vi "SendWait.vi"(0 "session in":refnum<k35>, 5 "Time (s)":i32, 7 "Text To Wait":string, 11 "error in":errorcluster) -> (4 "session out":refnum<k35>, 15 "error out":errorcluster)   [LabVIEW 2023]
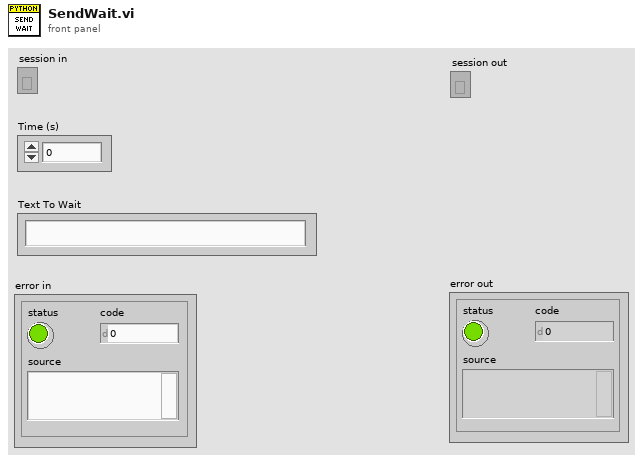
[diagram p1: front panel]
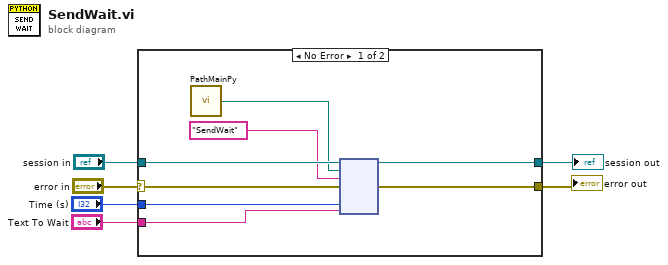
[diagram p0: block diagram]
diagram:
  n1 = case shown="No Error" "error in" {
    selector: "error in" -> [w11 w15]
    tunnel: "session in" -> [w14 w16]
    tunnel: [w13 w16] -> w3
    tunnel: [w12 w15] -> w4
    tunnel: "Text To Wait" -> [w8 _]
    tunnel: "Time (s)" -> [w7 _]
    frame No Error {
      n2 = call "PathMainPy.vi"() -> ("path"=w10:path)  [unwired: 15 in]
      n3 = node(w14, w10, "SendWait" ("function name"), w11, w7, w8) -> (w13:refnum<k35>, w12:errorcluster)  [unwired: 4 in, 2 out]
    }
    frame Error {
    }
  }
  "error out" <- w4
  "session out" <- w3
